vi "Core Test.vi"() -> ()   [LabVIEW 2019]
doc: "Tests the Quick Format Core VI by affecting the Test Target VI."
uses:
  Quick Format QD.lvlib
panel:
  in  "Format String":string
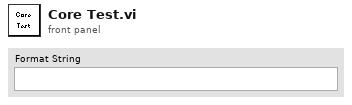
[diagram p1: front panel]
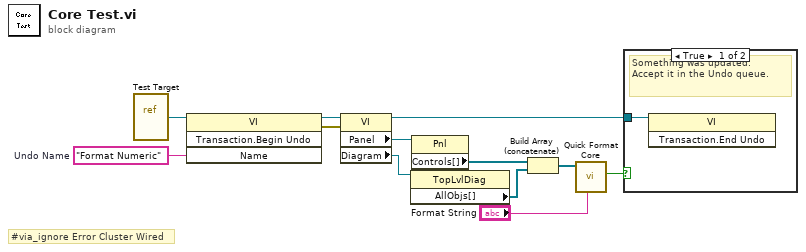
[diagram p0: block diagram]
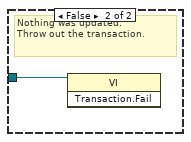
[diagram p2: hidden frame]
diagram:
  w5 = "Format Numeric"  # Undo Name
  # "#via_ignore Error Cluster Wired"
  n1 = vi-ref "Test Target.vi"() -> (w3:refnum<vi>)
  n2 = invoke class="VI" method="Transaction.Begin Undo"(reference=w3, "Name"=w5) -> (reference out=w4:refnum<vi>, error out=w12:errorcluster)  [unwired: 2 in, 2 out]
  n3 = property class="VI"(reference=w4, error in=w12) -> (reference out=w2:refnum<vi>, "Panel"=w11:refnum<vi>, "Diagram"=w10:refnum<vi>)  [unwired: 1 out]
  n4 = property class="TopLvlDiag"(reference=w10) -> ("AllObjs[]"=w8:refnum<vi>[])  [unwired: 1 in, 2 out]
  n5 = property class="Pnl"(reference=w11) -> ("Controls[]"=w9:refnum<vi>[])  [unwired: 1 in, 2 out]
  n6 = Build Array (concatenate)(w9, w8) -> (w7:refnum<vi>[])
  n7 = call "Quick Format Core.vi"("Format String"="Format String", "GObjects"=w7) -> ("Successful"=w1:bool)  [unwired: 9 in]
  n8 = case shown="True" w1 {
    tunnel: w2 -> [w13 w14]
    frame True {
      # "Something was updated.\nAccept it in the Undo queue."
      n9 = invoke class="VI" method="Transaction.End Undo"(reference=w13) -> ()  [unwired: 2 in, 3 out]
    }
    frame False {
      # "Nothing was updated.\nThrow out the transaction."
      n10 = invoke class="VI" method="Transaction.Fail"(reference=w14) -> ()  [unwired: 2 in, 3 out]
    }
  }
